vi "createCPETInstances.vi"(8 "error in (no error)":errorcluster, 11 "reference in":refnum<class "Devices Controller.lvclass">) -> (0 "error out":errorcluster, 3 "reference out":refnum<class "Devices Controller.lvclass">)   [LabVIEW 2016, in "Devices Controller.lvclass"]
uses:
  Devices Controller.lvclass
  deviceType.ctl
  APP/cpet_class/cpet.lvclass
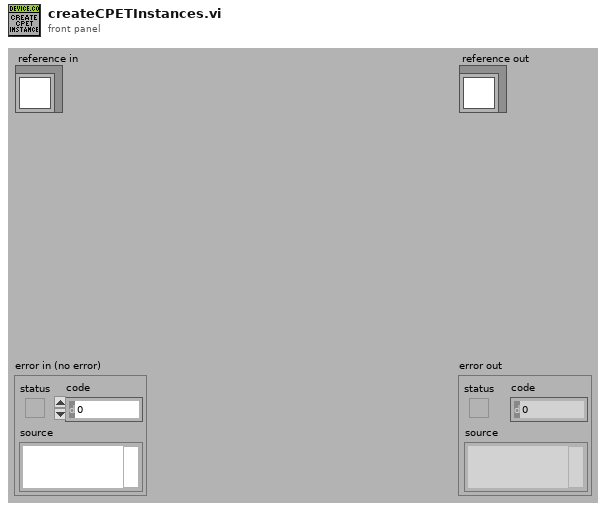
[diagram p1: front panel]
types:
  T1 = typedef "Devices Controller.lvclass/deviceType.ctl" = enum16{"k5", "k4b2", "fitmate", "cpet", "rmr", "bodyBoxPft", "bp", "pp"}
  T2 = typedef "Devices Controller.lvclass/ObjectAttributesRef.ctl" = refnum<data-value>
  T3 = typedef "Devices Controller.lvclass/ObjectAttributes.ctl" = cluster{"MyAttribute":dbl, "file_controller_ref":refnum<class "File Controller.lvclass">, "data":string[][][], "devices_refs":cluster{"k4b2_refs":refnum<class "k4b2.lvclass">[], "rmr_refs":refnum<class "rmr.lvclass">[], "bod_pod_refs":refnum<class "bodpod.lvclass">[], "cpet_refs":refnum<class "cpet.lvclass">[], "fitmate_refs":refnum<class "fitmate.lvclass">[], "pea_pod_refs":refnum<class "peapod.lvclass">[], "k5_refs":refnum<class "k5.lvclass">[], "bb-pft_refs":refnum<class "bb-pft.lvclass">[]}}
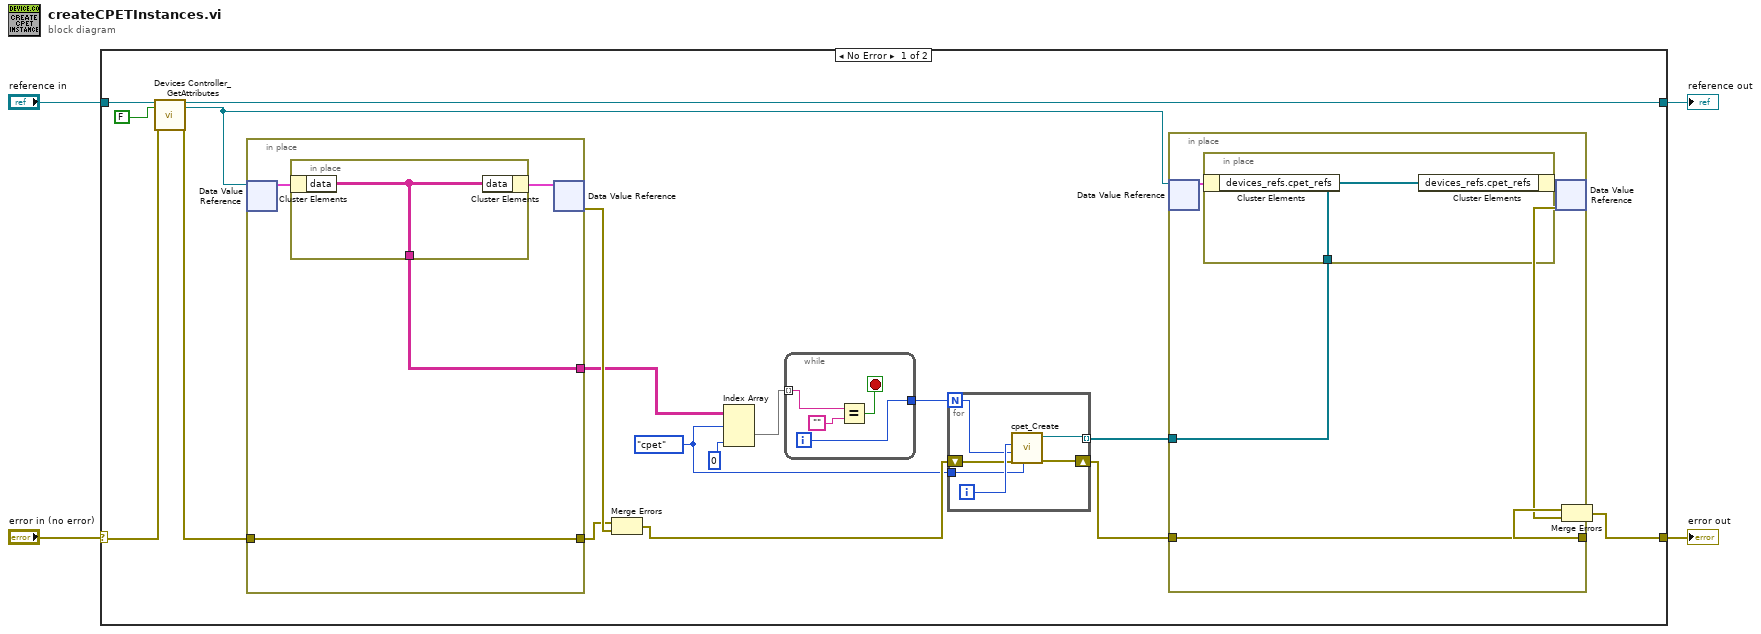
[diagram p0: block diagram]
diagram:
  n1 = case shown="No Error" "error in (no error)" {
    selector: "error in (no error)" -> [w19 w45]
    tunnel: [w10 w45] -> w3
    tunnel: [w17 w44] -> w1
    tunnel: "reference in" -> [w21 w44]
    frame No Error {
      w5 = deviceType."cpet" ("deviceType")
      n2 = call "Devices Controller_GetAttributes.vi"("reference in"=w21, "return data? (T)"=FALSE, "error in (no error)"=w19) -> ("reference out"=w17:refnum<class "Devices Controller.lvclass">, "attributes ref"=w9:T2, "error out"=w18:errorcluster)  [unwired: 13 in, 1 out]
      n3 = in-place {
        in-place-border: w18 -> [w40]
        in-place-border: [w40] -> w22
        in-place-border: [w39] -> w16
        n4 = in-place-dvr #1(w9) -> (w41:T3)  [unwired: 1 out]
        n5 = in-place {
          in-place-border: [w43] -> w39
          n6 = in-place-cluster #2(w41) -> ("data"=w43:string[][][])
          n7 = in-place-cluster #2("data"=w43) -> (w42:T3)
        }
        n8 = in-place-dvr #1(w42) -> (w23:errorcluster)  [unwired: 1 out]
      }
      n9 = Merge Errors(w22, w23) -> (w14:errorcluster)
      n10 = Index Array(array=w16, index (dim 0)=w5, index (dim 2)=0 ("index (row)")) -> (element=w7:string[])  [unwired: 1 in]
      n11 = while {
        tunnel: w7 -> [w27] mode=indexing
        tunnel: [w24] -> w6
        i -> [w24]
        stop <- w25 stop-if-true
        n12 = Equal?(x=w27, y="") -> (x = y?=w25:bool)
      }
      n13 = for {
        N: w6 -> [w35]
        shift-right: [w37] -> w13
        shift-left: w14 -> [w36]
        tunnel: w5 -> [w34]
        tunnel: [w33] -> w8 mode=indexing
        i -> [w38]
        n14 = call "cpet_Create.vi"("deviceType"=w34, "error in (no error)"=w36, "dim"=w35, "index"=w38) -> ("error out"=w37:errorcluster, "reference out"=w33:refnum<class "cpet.lvclass">)  [unwired: 6 in]
      }
      n15 = in-place {
        in-place-border: w13 -> [w29]
        in-place-border: [w29] -> w12
        in-place-border: w8 -> [w28]
        n16 = in-place-dvr #3(w9) -> (w30:T3)  [unwired: 1 out]
        n17 = in-place {
          in-place-border: w28 -> [w32]
          n18 = in-place-cluster #4(w30) -> ()  [unwired: 1 out]
          n19 = in-place-cluster #4("devices_refs.cpet_refs"=w32) -> (w31:T3)
        }
        n20 = in-place-dvr #3(w31) -> (w11:errorcluster)  [unwired: 1 out]
      }
      n21 = Merge Errors(w12, w11) -> (w10:errorcluster)
    }
    frame Error {
    }
  }
  "error out" <- w3
  "reference out" <- w1
